vi "Delete Node From Dictionary.vi"(8 "error in (no error)":errorcluster, 10 "UID":string, 11 "Base Tree in":refnum<class "Base Tree.lvclass">) -> (0 "error out":errorcluster, 3 "Base Tree out":refnum<class "Base Tree.lvclass">)   [LabVIEW 2017, in "Browser Core.lvlib" / "Base Tree.lvclass"]
doc: "Remove Node Class and Name pair from dictionary"
uses:
  Base Tree.lvclass
  Base Tree.lvclass/Base Tree.ctl
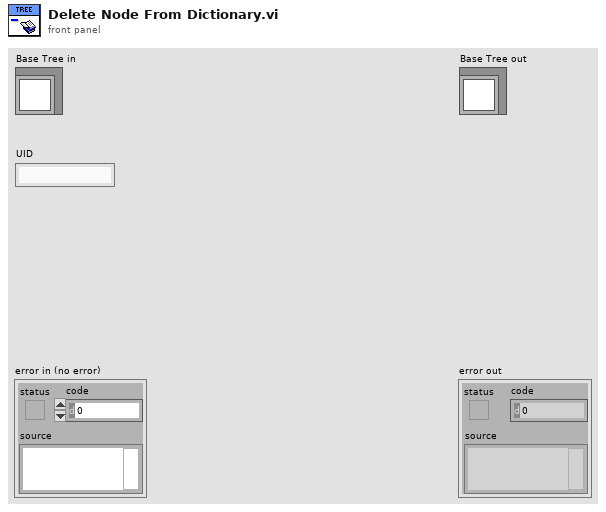
[diagram p1: front panel]
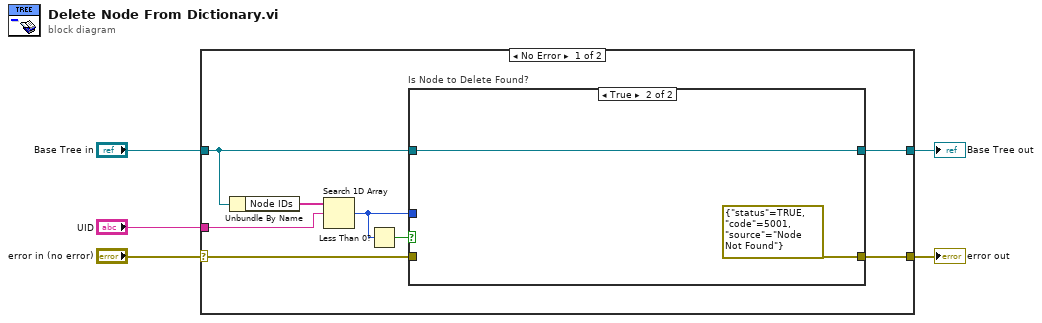
[diagram p0: block diagram]
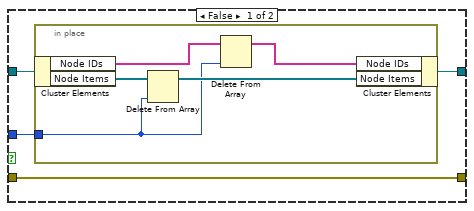
[diagram p2: hidden frame]
diagram:
  n1 = case shown="No Error" "error in (no error)" {
    selector: "error in (no error)" -> [w11 w26]
    tunnel: [w7 w26] -> w4
    tunnel: [w6 w25] -> w2
    tunnel: "Base Tree in" -> [w8 w25]
    tunnel: "UID" -> [w12 _]
    frame No Error {
      n2 = Unbundle By Name(w8) -> ("Node IDs"=w13:string[])
      n3 = Search 1D Array(1D array=w13, element=w12) -> (index of element=w9:i32)  [unwired: 1 in]
      n4 = Less Than 0?(x=w9) -> (x < 0?=w10:bool)
      n5 = case "Is Node to Delete Found?" shown="True" w10 {
        tunnel: w11 -> [w17 _]
        tunnel: w9 -> [w15 _]
        tunnel: w8 -> [w16 w23]
        tunnel: [w17 errorcluster {"status"=TRUE, "code"=5001, "source"="Node Not Found"} ("error IO")] -> w7
        tunnel: [w14 w23] -> w6
        frame False {
          n6 = in-place {
            in-place-border: w15 -> [w19]
            n7 = in-place-cluster #1(w16) -> ("Node IDs"=w21:string[], "Node Items"=w22:refnum<class "Generic Node.lvclass">[])
            n8 = Delete From Array(array=w22, index=w19) -> (array with subset deleted=w20:refnum<class "Generic Node.lvclass">[])  [unwired: 1 in, 1 out]
            n9 = Delete From Array(array=w21, index=w19) -> (array with subset deleted=w18:string[])  [unwired: 1 in, 1 out]
            n10 = in-place-cluster #1("Node IDs"=w18, "Node Items"=w20) -> (w14:refnum<class "Base Tree.lvclass">)
          }
        }
        frame True {
        }
      }
    }
    frame Error {
      # "Do Not Change Private Data On Error In"
    }
  }
  "error out" <- w4
  "Base Tree out" <- w2
